vi "layout.vi"(0 "reference":refnum<class "InterfaceNode.lvclass">, 1 "graph":refnum<class "Graph.lvclass">, 2 "graphics":refnum<class "Graphics.lvclass">, 3 "grid":refnum<class "Grid.lvclass">, 5 "error in (no error)":errorcluster) -> (14 "reference out":refnum<class "InterfaceNode.lvclass">, 19 "error out":errorcluster)   [LabVIEW 2020, in "InterfaceNode.lvclass"]
doc: "public void layout(Graph g, Graphics2D g2, Grid grid)"
uses:
  <resource>/Framework/Providers/Open_GDS/UML/InterfaceNode_class/InterfaceNode.lvclass
  <resource>/Framework/Providers/Open_GDS/UML/Graph_class/Graph.lvclass
  <resource>/Framework/Providers/Open_GDS/UML/Graphics_class/Graphics.lvclass
  <resource>/Framework/Providers/Open_GDS/UML/Grid_class/Grid.lvclass
  <resource>/Framework/Providers/Open_GDS/UML/ClassNode_class/ClassNode.lvclass
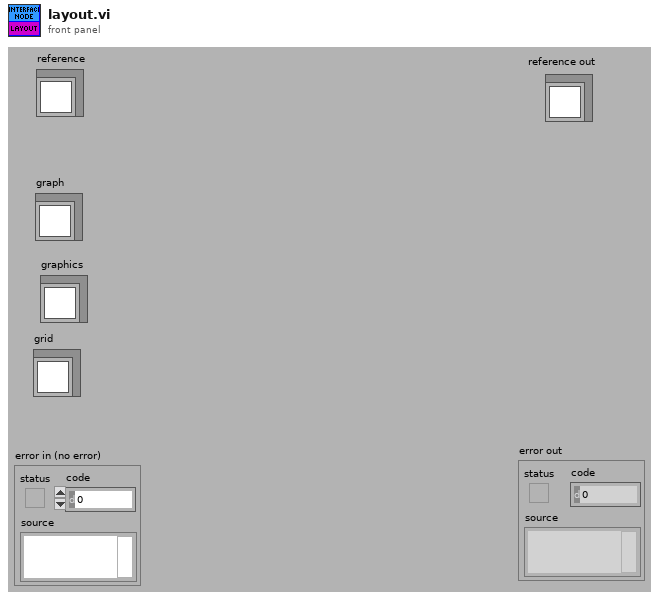
[diagram p1: front panel]
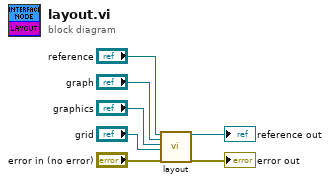
[diagram p0: block diagram]
diagram:
  n1 = call-parent "layout.vi"("reference"="reference", "graph"="graph", "graphics"="graphics", "grid"="grid", "error in (no error)"="error in (no error)") -> ("reference out"=→"reference out":refnum<class "InterfaceNode.lvclass">, "error out"=→"error out":errorcluster)  [unwired: 13 in]
